vi "Sweep Reset WL Test.vi"(8 "error in (no error)":errorcluster, 9 "Sweep outfile":path, 10 "addr":i32, 11 "instrument handle":refnum<k15>) -> (0 "error out":errorcluster, 1 "final current (A)":dbl, 2 "final resistance (ohm)":dbl, 3 "instrument handle out":refnum<k15>)   [LabVIEW 2018]
uses:
  <instrlib>/niDigital/niDigital.llb/niDigital Burst Pattern (Burst Only).vi
  <vilib>/Utility/file.llb/Write Delimited Spreadsheet (DBL).vi
panel:
  out "i":i32
  out "PW":dbl
  out "BL voltage (V)":dbl
  out "WL voltage (V)":dbl
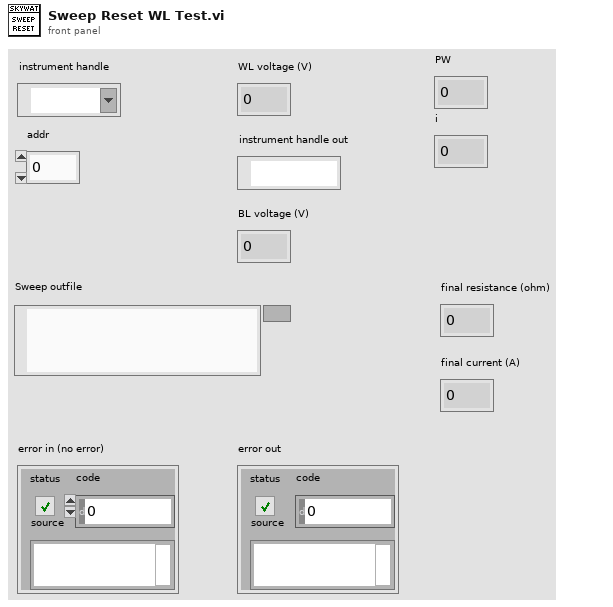
[diagram p1: front panel]
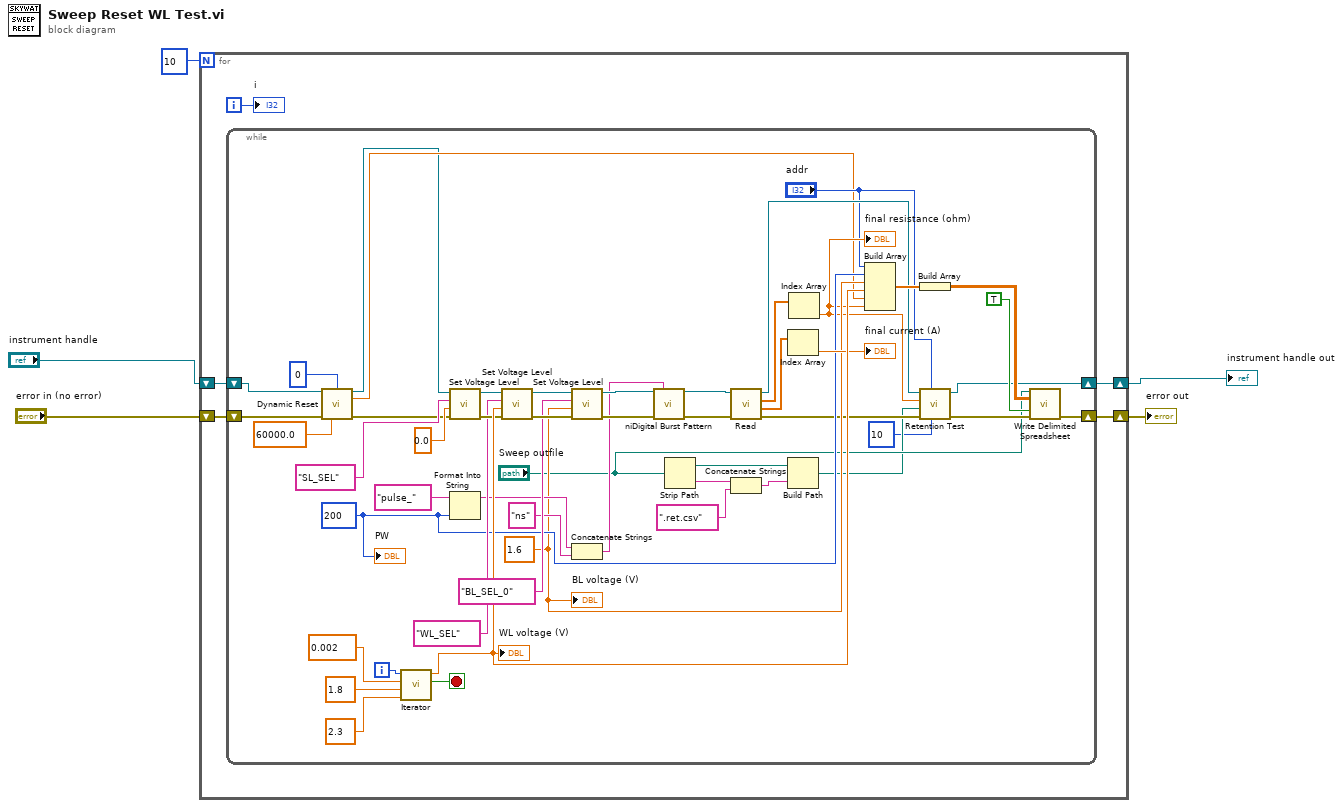
[diagram p0: block diagram]
diagram:
  n1 = for {
    N: 10 -> [_]
    shift-right: [w10] -> w5
    shift-left: "instrument handle" -> [w6]
    shift-right: [w9] -> w4
    shift-left: "error in (no error)" -> [w7]
    i -> [w8]
    n2 = while {
      shift-right: [w28] -> w10
      shift-left: w6 -> [w11]
      shift-right: [w58] -> w9
      shift-left: w7 -> [w14]
      i -> [w59]
      stop <- w55 stop-if-true
      w31 = 1.6 ("BL voltage (V)")
      w32 = 200 ("y")
      n3 = call "Dynamic Reset.vi"("instrument handle"=w11, "index"=0, "error in (no error)"=w14, "target resistance (ohm)"=60000.0) -> ("instrument handle out"=w12:refnum<k15>, "final resistance (ohm)"=w15:dbl, "error out"=w13:errorcluster)  [unwired: 5 in, 4 out]
      n4 = call "Iterator.vi"("Final Value"=2.3 ("y"), "Initial Value"=1.8 ("y"), "Step"=0.002 ("x"), "i"=w59) -> ("End Loop"=w55:bool, "Current Value"=w56:dbl)  [unwired: 6 in]
      "WL voltage (V)" <- w56
      n5 = call "Set Voltage Level.vi"("error in (no error)"=w13, "level (V)"=0.0, "channel list"="SL_SEL", "instrument handle"=w12) -> ("error out"=w51:errorcluster, "instrument handle out"=w52:refnum<k15>)  [unwired: 6 in]
      n6 = Format Into String(initial string="pulse_" ("start label"), w32) -> (resulting string=w34:string)  [unwired: 2 in, 1 out]
      n7 = call "Set Voltage Level.vi"("error in (no error)"=w51, "level (V)"=w56, "channel list"="WL_SEL", "instrument handle"=w52) -> ("error out"=w54:errorcluster, "instrument handle out"=w53:refnum<k15>)  [unwired: 6 in]
      n8 = call "Set Voltage Level.vi"("error in (no error)"=w54, "level (V)"=w31, "channel list"="BL_SEL_0", "instrument handle"=w53) -> ("error out"=w46:errorcluster, "instrument handle out"=w45:refnum<k15>)  [unwired: 6 in]
      n9 = Concatenate Strings(w34, "ns" ("string")) -> (w33:string)
      n10 = call-poly <instrlib>:"niDigital Burst Pattern.vi"("instrument handle"=w45, "start label"=w33, "error in"=w46) -> ("instrument handle out"=w40:refnum<k15>, "error out"=w41:errorcluster)  [unwired: 11 in]
      n11 = Strip Path(path="Sweep outfile") -> (stripped path=w20:path, name=w24:string)
      n12 = call "Read.vi"("error in (no error)"=w41, "instrument handle"=w40) -> ("error out"=w26:errorcluster, "currents (A)"=w38:dbl[], "resistances (ohm)"=w39:dbl[], "instrument handle out"=w29:refnum<k15>)  [unwired: 6 in]
      n13 = Concatenate Strings(w24, ".ret.csv" ("string")) -> (w22:string)
      n14 = Index Array(array=w38) -> (element=→"final current (A)":dbl)  [unwired: 1 in]
      n15 = Build Path(base path=w20, name or relative path=w22) -> (appended path=w19:path)
      n16 = Index Array(array=w39) -> (element=w30:dbl)  [unwired: 1 in]
      "final resistance (ohm)" <- w30
      n17 = Build Array("addr", w32, w31, w56, w15, w30) -> (w43:dbl[])
      n18 = Build Array(w43) -> (w44:dbl[][])
      n19 = call "Retention Test.vi"("Reads"=10, "Current address"="addr", "error in (no error)"=w26, "target outfile"=w19, "final resistance (ohm)"=w30, "IVI Refnum in"=w29) -> ("error out"=w25:errorcluster, "IVI Refnum out"=w28:refnum<k15>)  [unwired: 4 in]
      n20 = call-poly <vilib>:"Write Delimited Spreadsheet.vi"("file path (dialog if empty)"="Sweep outfile", "2D data"=w44, "append to file? (new file:F)"=TRUE, "error in (no error)"=w25) -> ("error out"=w58:errorcluster)  [unwired: 10 in, 1 out]
      "BL voltage (V)" <- w31
      "PW" <- w32
    }
    "i" <- w8
  }
  "error out" <- w4
  "instrument handle out" <- w5
